vi "APC_9056_RT_main.vi"   [LabVIEW 2020]
panel:
  # "monarch APC v0.1"
  # "cRIO 9056 RT main"
types:
  T1 = cluster{"Queue array":dbl[], "Channel list":string[], "TS queue":refnum<queue>, "TS signals path":string}
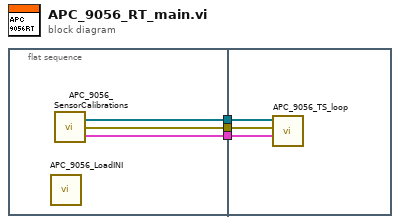
[diagram p0: block diagram]
diagram:
  n1 = flat-sequence {
    tunnel: [w6] -> w3
    tunnel: [w5] -> w2
    tunnel: [w4] -> w1
    tunnel: w3 -> [w9]
    tunnel: w2 -> [w8]
    tunnel: w1 -> [w7]
    frame #0 {
      n2 = call "APC_9056_LoadINI.vi"() -> ()  [unwired: 4 in]
      n3 = call "APC_9056_SensorCalibrations.vi"() -> ("DAQqueue"=w4:T1, "error out"=w5:errorcluster, "DAQmx I tasks"=w6:refnum<k21>[])
    }
    frame #1 {
      n4 = call "APC_9056_TS_loop.vi"("DAQqueue"=w7, "error in"=w8, "scaled dAQmx task"=w9) -> ()  [unwired: 1 in]
    }
  }
